vi "Draw Rectangle XY Graph.vi"(7 "rect":T1={"left"=10.0, "top"=55.0, "right"=110.0, "bottom"=5.0}) -> (8 "XY Graph Out":cluster{dbl[], dbl[]}(graph))   [LabVIEW 2014]
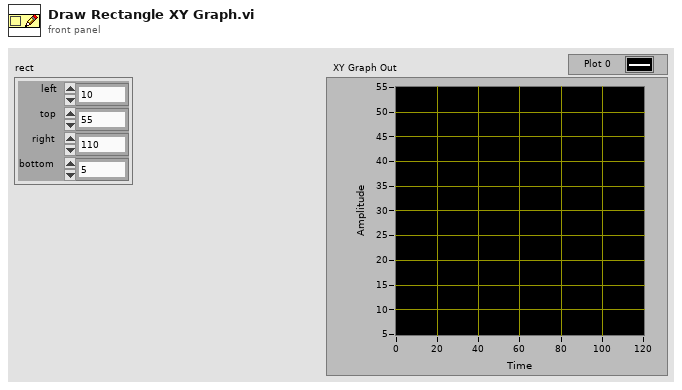
[diagram p1: front panel]
types:
  T1 = cluster{"left":dbl, "top":dbl, "right":dbl, "bottom":dbl}
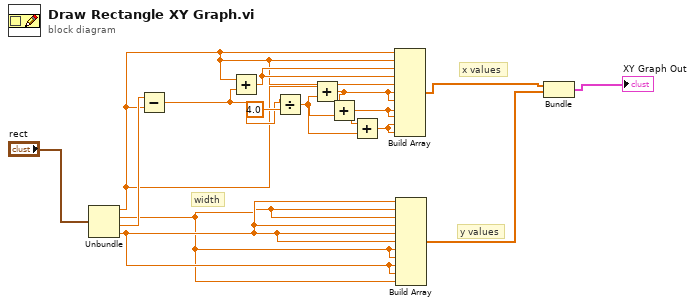
[diagram p0: block diagram]
diagram:
  # "y values"
  # "x values"
  # "width"
  n1 = Unbundle("rect") -> ("left"=w3:dbl, "top"=w5:dbl, "right"=w13:dbl, "bottom"=w8:dbl)
  n2 = Subtract(x=w13, y=w3) -> (x-y=w4:dbl)
  n3 = Add(x=w3, y=w4) -> (x+y=w14:dbl)
  n4 = Divide(x=w4, y=4.0) -> (x/y=w2:dbl)
  n5 = Add(x=w3, y=w2) -> (x+y=w1:dbl)
  n6 = Add(x=w1, y=w2) -> (x+y=w7:dbl)
  n7 = Add(x=w7, y=w2) -> (x+y=w6:dbl)
  n8 = Build Array(w3, w3, w14, w14, w3, w1, w1, w7, w7, w6, w6) -> (w12:dbl[])
  n9 = Build Array(w8, w5, w5, w8, w8, w8, w5, w5, w8, w8, w5) -> (w11:dbl[])
  n10 = Bundle(w12, w11) -> (→"XY Graph Out":cluster{dbl[], dbl[]})  [unwired: 1 in]
